vi "Make Zero Vector.vi"(11 "Columns":i32) -> (2 "Zero Vector":T1)   [LabVIEW 2009]
uses:
  <vilib>/Analysis/Matrix/Datatypes/RealMatrix.ctl
  <vilib>/Analysis/Matrix/NI_Matrix.lvlib
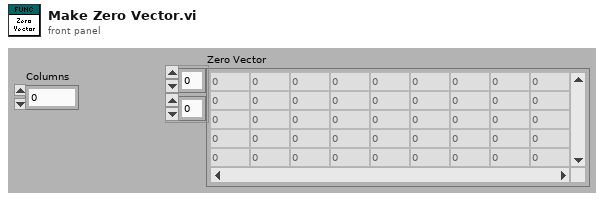
[diagram p1: front panel]
types:
  T1 = typedef "NI_Matrix.lvlib/RealMatrix.ctl" = dbl[][]
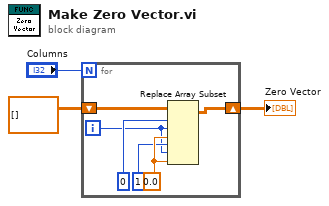
[diagram p0: block diagram]
diagram:
  n1 = for {
    N: "Columns" -> [_]
    shift-right: [w8] -> w1
    shift-left: T1 [] ("matrix") -> [w9]
    i -> [w4]
    w6 = 0.0 ("new element/submatrix")
    n2 = Replace Array Subset(array=w9, new element #1=w6, index (row) #1=0 ("disabled index (row)"), index (col) #1=w4, new element #2=w6, index (row) #2=1 ("disabled index (row)"), index (col) #2=w4) -> (w8:T1)
  }
  "Zero Vector" <- w1
